vi "Convert Numeric Array Key Value Pairs to Log Rows.vi"(8 "error in (no error)":errorcluster, 9 "Data[]":string[](array[string])=["1", "", "3"], 10 "Numeric Array Key Value Pairs":cluster{"Key":string, "Value":dbl[]}[](array[cluster])=[{"Key"="Header 2", "Value"=[21.0, 22.0]}], 11 "Headers In[]":string[](array[string])=["Header 1", "Header 2", "Header 3"]) -> (0 "error out":errorcluster, 3 "Log Data[][]":string[][](array[string]))   [LabVIEW 2016, in "SLL Spreadsheet.lvlib" / "SLL CSV Logger.lvclass"]
uses:
  SLL CSV Logger.lvclass
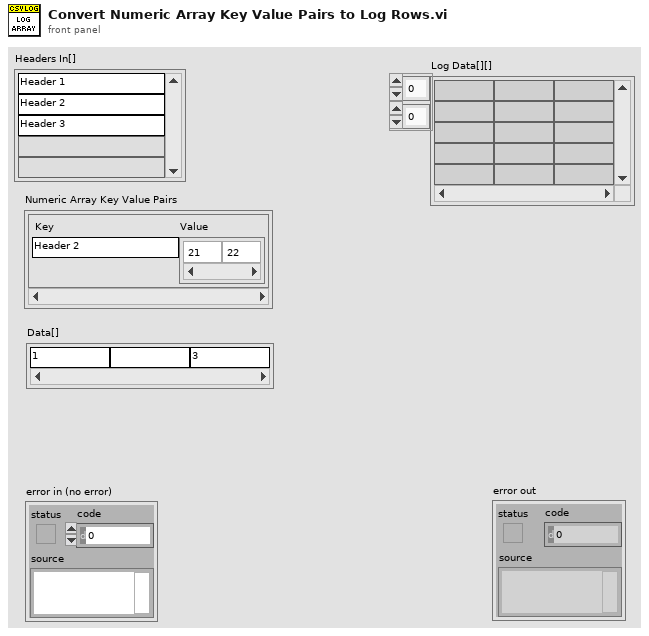
[diagram p1: front panel]
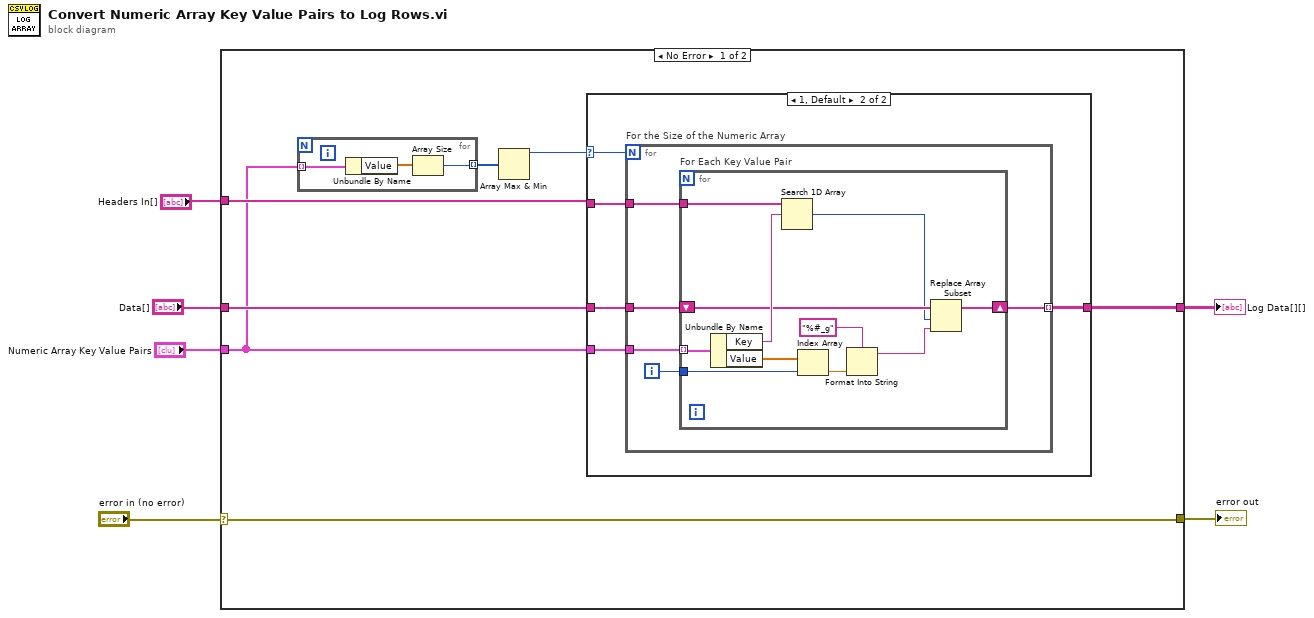
[diagram p0: block diagram]
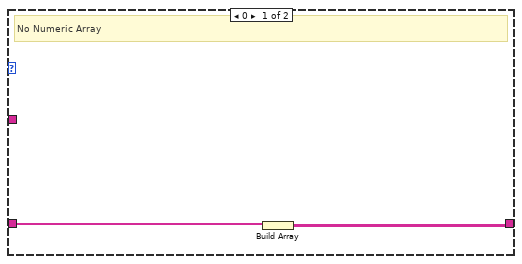
[diagram p2: hidden frame]
diagram:
  n1 = case shown="No Error" "error in (no error)" {
    selector: "error in (no error)" -> [w13 w40]
    tunnel: [w13 w40] -> w5
    tunnel: "Headers In[]" -> [w11 _]
    tunnel: "Numeric Array Key Value Pairs" -> [w9 _]
    tunnel: "Data[]" -> [w12 _]
    tunnel: [w10 _] -> w1
    frame No Error {
      n2 = for {
        tunnel: [w15] -> w8 mode=indexing
        tunnel: w9 -> [w14] mode=indexing
        n3 = Unbundle By Name(w14) -> ("Value"=w16:dbl[])
        n4 = Array Size(array=w16) -> (size(s)=w15:i32)
      }
      n5 = Array Max & Min(array=w8) -> (max value=w7:i32)  [unwired: 3 out]
      n6 = case shown="1, Default" w7 {
        selector: w7 -> [_ w19]
        tunnel: w12 -> [w18 w23]
        tunnel: w11 -> [_ w22]
        tunnel: [w17 w21] -> w10
        tunnel: w9 -> [_ w20]
        frame 0 {
          # "No Numeric Array"
          n7 = Build Array(w18) -> (w17:string[][])
        }
        frame 1, Default {
          n8 = for "For the Size of the Numeric Array" {
            N: w19 -> [_]
            tunnel: w23 -> [w27]
            tunnel: w20 -> [w26]
            tunnel: w22 -> [w28]
            tunnel: [w24] -> w21 mode=indexing
            i -> [w25]
            n9 = for "For Each Key Value Pair" {
              tunnel: w28 -> [w38]
              tunnel: w26 -> [w39] mode=indexing
              tunnel: w25 -> [w34]
              shift-right: [w29] -> w24
              shift-left: w27 -> [w36]
              n10 = Unbundle By Name(w39) -> ("Key"=w37:string, "Value"=w35:dbl[])
              n11 = Search 1D Array(1D array=w38, element=w37) -> (index of element=w31:i32)  [unwired: 1 in]
              n12 = Index Array(array=w35, index=w34) -> (element=w33:dbl)
              n13 = Format Into String(format string="%#_g", w33) -> (resulting string=w30:string)  [unwired: 2 in, 1 out]
              n14 = Replace Array Subset(array=w36, new element=w30, index=w31) -> (w29:string[])
            }
          }
        }
      }
    }
    frame Error {
    }
  }
  "error out" <- w5
  "Log Data[][]" <- w1
